vi "New.vi"(8 "error in (no error)":errorcluster, 10 "niVI":string, 11 "Image":T1) -> (0 "error out":errorcluster, 3 "VI Snippet out":T2)   [LabVIEW 2022 SP3, in "VI-Snippet.lvlib"]
doc: "Creates a new Snippet instance."
uses:
  VI-Snippet.lvlib
  Snippet.ctl
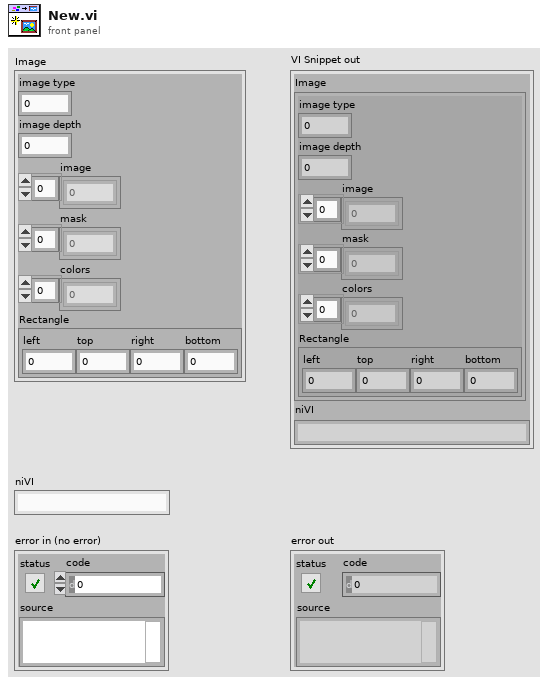
[diagram p1: front panel]
types:
  T1 = cluster{"image type":i32, "image depth":i32, "image":u8[], "mask":u8[], "colors":u32[], "Rectangle":cluster{"left":i16, "top":i16, "right":i16, "bottom":i16}}
  T2 = typedef "VI-Snippet.lvlib/Snippet.ctl" = cluster{"Image":cluster{"image type":i32, "image depth":i32, "image":u8[], "mask":u8[], "colors":u32[], "Rectangle":cluster{"left":i16, "top":i16, "right":i16, "bottom":i16}}, "niVI":string}
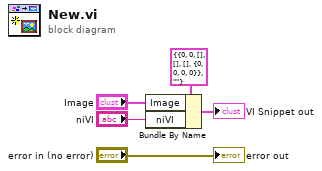
[diagram p0: block diagram]
diagram:
  n1 = Bundle By Name(cluster=T2 {"Image"={"image type"=0, "image depth"=0, "image"=[], "mask"=[], "colors"=[], "Rectangle"={"left"=0, "top"=0, "right"=0, "bottom"=0}}, "niVI"=""} ("VI Snippet in"), "Image"="Image", "niVI"="niVI") -> (→"VI Snippet out":T2)
  "error out" <- "error in (no error)"
